vi "GetOperationInstrumentSMURegister.vi"(7 "SMU":T2, 8 "Error In":errorcluster, 10 "Register":T1, 11 "Kiethley 2602 In":refnum<visa-resource-name>) -> (0 "Error Out":errorcluster, 2 "Operation Instrument SMU Register":bool[](array[boolean]), 3 "Keithley 2602 Out":refnum<visa-resource-name>)   [LabVIEW 2012, in "Keithley-2602.lvlib"]
uses:
  Keithley-2602.lvlib
  Controls/SMU.ctl
  Controls/Register.ctl
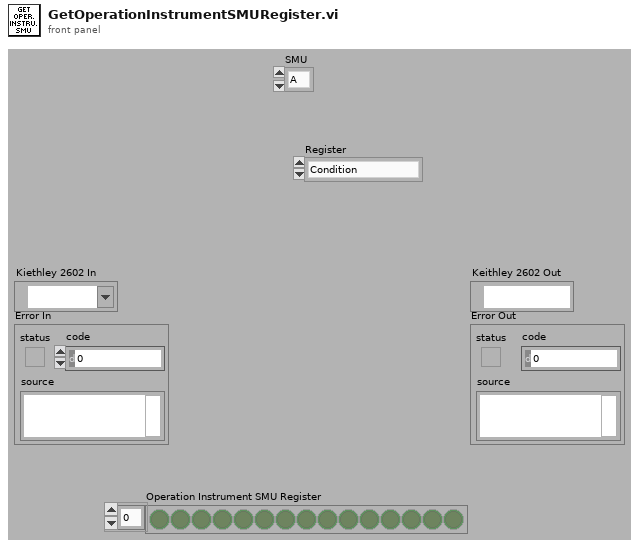
[diagram p1: front panel]
types:
  T1 = typedef "Keithley-2602.lvlib/Register.ctl" = enum16{"Condition", "Event", "Enable", "Positive Transition", "Negative Transition"}
  T2 = typedef "Keithley-2602.lvlib/SMU.ctl" = enum16{"A", "B"}
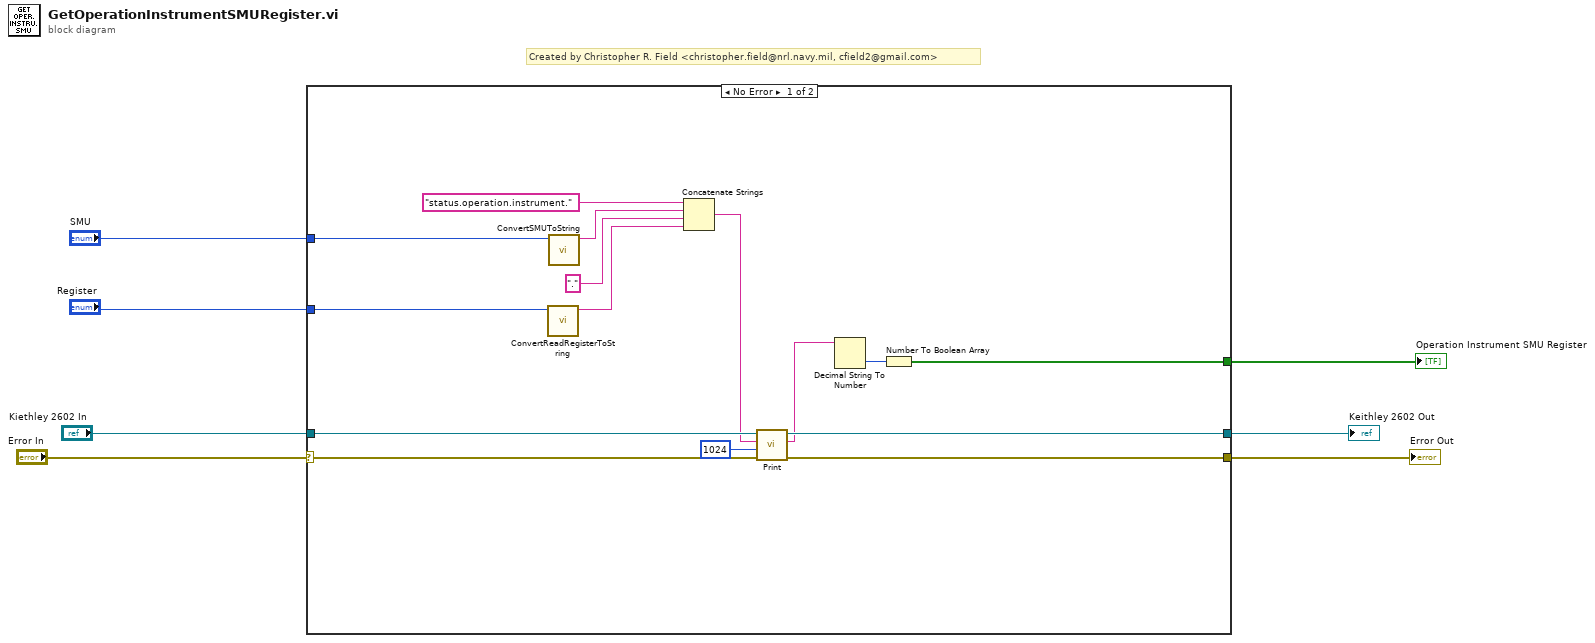
[diagram p0: block diagram]
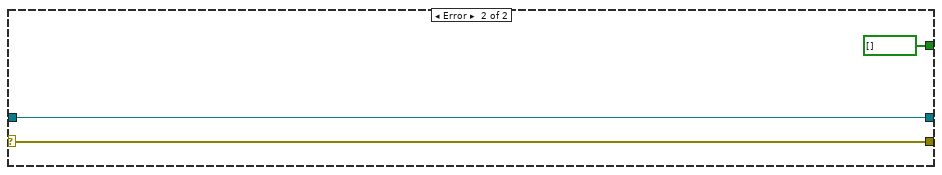
[diagram p2: hidden frame]
diagram:
  # "Created by Christopher R. Field <christopher.field@nrl.navy.mil, cfield2@gmail.com>"
  n1 = case shown="No Error" "Error In" {
    selector: "Error In" -> [w8 w25]
    tunnel: "Kiethley 2602 In" -> [w22 w24]
    tunnel: [w20 w24] -> w6
    tunnel: [w19 w25] -> w5
    tunnel: [w16 bool[] [] ("Boolean array")] -> w4
    tunnel: "SMU" -> [w10 _]
    tunnel: "Register" -> [w9 _]
    frame No Error {
      n2 = call "ConvertReadRegisterToString.vi"("Register"=w9) -> ("Register"=w12:string)  [unwired: 10 in]
      n3 = call "ConvertSMUToString.vi"("SMU"=w10) -> ("Channel"=w14:string)  [unwired: 10 in]
      n4 = Concatenate Strings("status.operation.instrument.", w14, "." ("string"), w12) -> (w11:string)
      n5 = call "Print.vi"("Error In"=w8, "Byte Count"=u32 1024, "Attribute"=w11, "Kiethley 2602 In"=w22) -> ("Error Out"=w19:errorcluster, "Output"=w18:string, "Keithley 2602 Out"=w20:refnum<visa-resource-name>)  [unwired: 5 in]
      n6 = Decimal String To Number(string=w18) -> (number=w17:i32)  [unwired: 2 in, 1 out]
      n7 = Number To Boolean Array(number=w17) -> (Boolean array=w16:bool[])
    }
    frame Error {
    }
  }
  "Keithley 2602 Out" <- w6
  "Error Out" <- w5
  "Operation Instrument SMU Register" <- w4
